vi "From SettingsCluster To SpecificCluster.vi"(0 "variant  (source)":variant=variant(cluster{"resourcename":string, "Trigger":enum16{"off", "on"}, "timeout":cluster{"Value":dbl, "Min":dbl, "Max":dbl, "StepSize":dbl, "Tolerance":dbl, "valueactual":dbl}, "LocalSavingPath":path, "Save":enum16{"off", "on"}, "channels":string, "probeattenuation":cluster{"Channel1":cluster{"Value":dbl, "Min":dbl, "Max":dbl, "StepSize":dbl, "Tolerance":dbl, "valueactual":dbl}, "Channel2":cluster{"Value":dbl, "Min":dbl, "Max":dbl, "StepSize":dbl, "Tolerance":dbl, "valueactual":dbl}}, "verticalrange":cluster{"Channel1":cluster{"Value":dbl, "Min":dbl, "Max":dbl, "StepSize":dbl, "Tolerance":dbl, "valueactual":dbl}, "Channel2":cluster{"Value":dbl, "Min":dbl, "Max":dbl, "StepSize":dbl, "Tolerance":dbl, "valueactual":dbl}}, "channelenabled":cluster{"Channel1":enum16{"off", "on"}, "Channel2":enum16{"off", "on"}}, "coupling":cluster{"Channel1":enum16{"AC", "DC", "Ground"}, "Channel2":enum16{"AC", "DC", "Ground"}}, "offset":cluster{"Channel1":cluster{"Value":dbl, "Min":dbl, "Max":dbl, "StepSize":dbl, "Tolerance":dbl, "valueactual":dbl}, "Channel2":cluster{"Value":dbl, "Min":dbl, "Max":dbl, "StepSize":dbl, "Tolerance":dbl, "valueactual":dbl}}, "Impedance":cluster{"Channel1":enum16{"1 mega ohm", "NA", "50 ohms"}, "Channel2":enum16{"1 mega ohm", "NA", "50 ohms"}}} {"resourcename"="PXI1Slot6", "Trigger"=enum."off", "timeout"={"Value"=1.0, "Min"=0.0, "Max"=5.0, "StepSize"=0.5, "Tolerance"=0.0, "valueactual"=0.0}, "LocalSavingPath"=path "c:/temp", "Save"=enum."off", "channels"="1,2", "probeattenuation"={"Channel1"={"Value"=1.0, "Min"=0.0, "Max"=10.0, "StepSize"=0.1, "Tolerance"=0.0, "valueactual"=0.0}, "Channel2"={"Value"=5.0, "Min"=0.0, "Max"=10.0, "StepSize"=0.1, "Tolerance"=0.0, "valueactual"=0.0}}, "verticalrange"={"Channel1"={"Value"=3.0, "Min"=0.001, "Max"=30.0, "StepSize"=0.01, "Tolerance"=30.0, "valueactual"=0.0}, "Channel2"={"Value"=4.0, "Min"=0.001, "Max"=30.0, "StepSize"=0.01, "Tolerance"=30.0, "valueactual"=0.0}}, "channelenabled"={"Channel1"=enum."on", "Channel2"=enum."off"}, "coupling"={"Channel1"=enum."DC", "Channel2"=enum."Ground"}, "offset"={"Channel1"={"Value"=0.0, "Min"=-5.0, "Max"=5.0, "StepSize"=0.01, "Tolerance"=0.0, "valueactual"=0.0}, "Channel2"={"Value"=3.0, "Min"=-5.0, "Max"=5.0, "StepSize"=0.01, "Tolerance"=0.0, "valueactual"=0.0}}, "Impedance"={"Channel1"=enum."50 ohms", "Channel2"=enum."50 ohms"}}), 1 "variant (destination)":variant=variant(cluster{"verticalrange":dbl, "probeattenuation":dbl, "offset":dbl, "channelenabled":bool, "coupling":enum16{"AC", "DC", "Ground"}} {"verticalrange"=0.0, "probeattenuation"=0.0, "offset"=0.0, "channelenabled"=FALSE, "coupling"=enum."AC"}), 5 "Command":string="setverticalrange", 7 "Args":string[](array[string])=["5.000000", ".Channel2"], 9 "Seperator (\"\")":string="Channel", 11 "error in (no error)":errorcluster, 12 "number of group elements (0)":i32) -> (4 "variant out":variant=variant(cluster{"verticalrange":dbl, "probeattenuation":dbl, "offset":dbl, "channelenabled":bool, "coupling":enum16{"AC", "DC", "Ground"}} {"verticalrange"=5.0, "probeattenuation"=5.0, "offset"=3.0, "channelenabled"=FALSE, "coupling"=enum."Ground"}), 6 "Command out":string, 8 "Arg":string, 10 "Seperator out":string="Channel2", 15 "error  out":errorcluster)   [LabVIEW 2011]
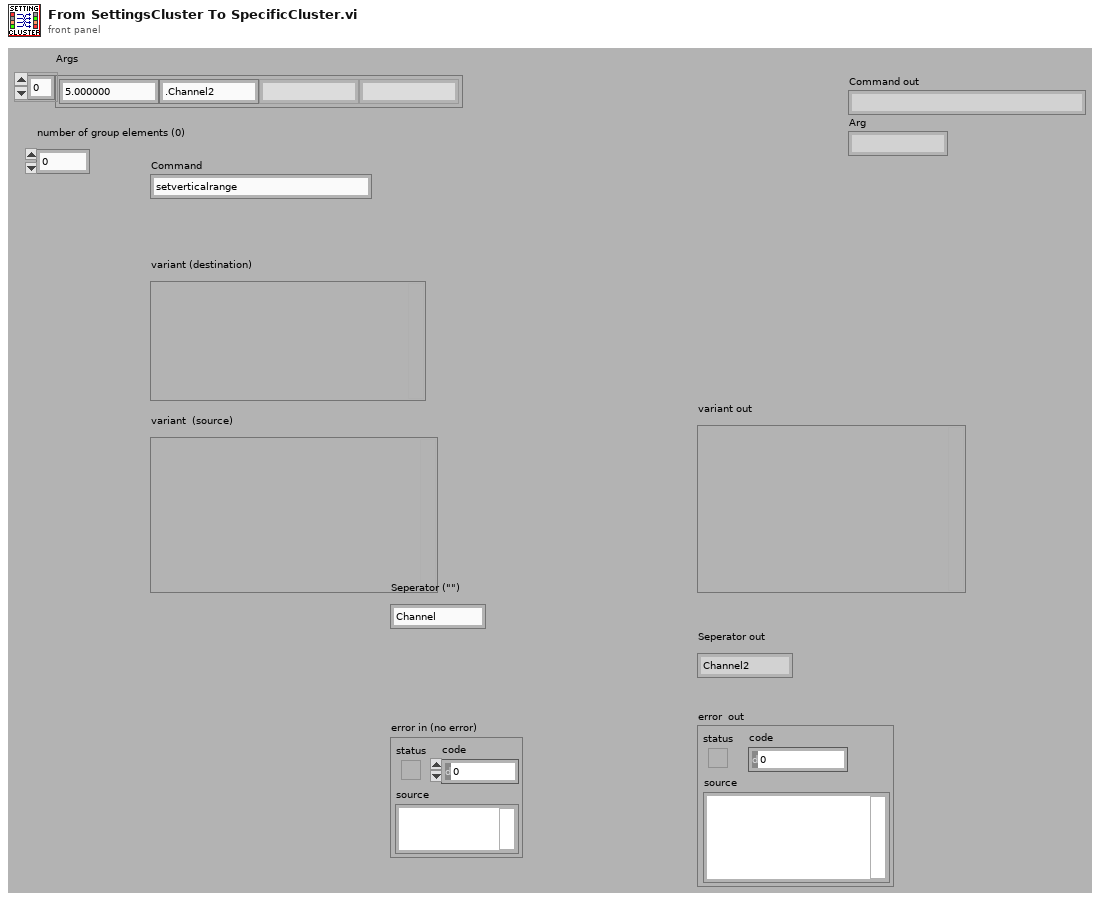
[diagram p1: front panel]
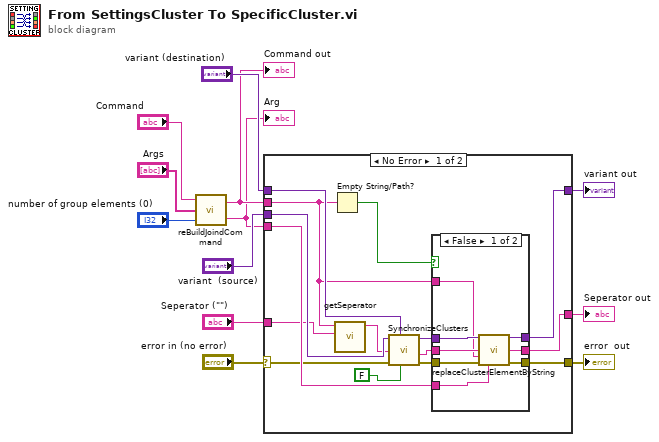
[diagram p0: block diagram]
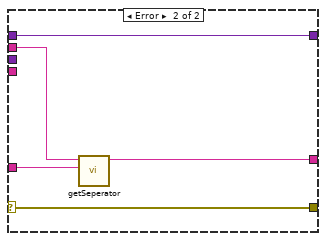
[diagram p3: hidden frame]
diagram:
  n1 = call "reBuildJoindCommand.vi"("number of group elements (0)"="number of group elements (0)", "Args"="Args", "Command 2"="Command") -> ("Arg"=w2:string, "Command"=w3:string)
  "Command out" <- w3
  "Arg" <- w2
  n2 = case shown="No Error" "error in (no error)" {
    selector: "error in (no error)" -> [w14 w43]
    tunnel: "variant  (source)" -> [w27 _]
    tunnel: "variant (destination)" -> [w26 w42]
    tunnel: [w24 w43] -> w11
    tunnel: [w22 w39] -> w10
    tunnel: [w21 w42] -> w6
    tunnel: w2 -> [w20 _]
    tunnel: "Seperator (\"\")" -> [w19 w40]
    tunnel: w3 -> [w17 w41]
    frame No Error {
      n3 = Empty String/Path?(string/path=w17) -> (empty?=w16:bool)
      n4 = call "getSeperator.vi"("Channel Seperator (\"\")"=w19, "Command"=w17) -> ("Seperator (e.g. \"Channel1\")"=w18:string)  [unwired: 8 in, 1 out]
      n5 = call "SynchronizeClusters.vi"("toSettings"=FALSE, "variant (destination)"=w26, "error in (no error)"=w14, "Seperator (\"\")"=w18, "variant  (source)"=w27) -> ("error  out"=w25:errorcluster, "Seperator out"=w23:string, "variant out"=w13:variant)  [unwired: 4 in]
      n6 = case shown="False" w16 {
        tunnel: w13 -> [w35 w38]
        tunnel: w25 -> [w34 w36]
        tunnel: [w33 w36] -> w24
        tunnel: w23 -> [w32 w37]
        tunnel: [w31 w37] -> w22
        tunnel: [w30 w38] -> w21
        tunnel: w20 -> [w29 _]
        tunnel: w17 -> [w28 _]
        frame False {
          n7 = call "replaceClusterElementByString.vi"("cluster in"=w35, "Seperator (\"\")"=w32, "Command"=w28, "error in (no error)"=w34, "setvalue"=w29) -> ("cluster out"=w30:variant, "Seperator (\"\") out"=w31:string, "error out"=w33:errorcluster)  [unwired: 8 in]
        }
        frame True {
        }
      }
    }
    frame Error {
      n8 = call "getSeperator.vi"("Channel Seperator (\"\")"=w40, "Command"=w41) -> ("Seperator (e.g. \"Channel1\")"=w39:string)  [unwired: 8 in, 1 out]
    }
  }
  "error  out" <- w11
  "Seperator out" <- w10
  "variant out" <- w6
